vi "Aux TE Controllers Initialization.vi"(8 "Error In":errorcluster, 9 "input cluster":T1={"Loaded Settings File"=path "", "Test Settings"={"Dual Channel"=FALSE, "Air Pump"=FALSE, "Optical Drive"=FALSE, "Pulsed Drive"=FALSE, "Calibration Mode"=FALSE, "Test Sensor ID"=0, "Test Chamber"="", "Test Operator"="", "Sample Descriptor"="", "Notes"=""}, "Calibration Settings"={"Cal. Average"=2, "Cal Averaging"=FALSE, "Tolerance #0"=0.0, "Tolerance #7"=0.0, "Tolerance #6"=0.0, "Tolerance #5"=0.0, "Tolerance #4"=0.0, "Tolerance #3"=0.0, "Tolerance #2"=0.0, "Tolerance #1"=0.0, "Gas Tank Settings"={"Gas Conc. #0"="", "Gas Conc. #1"=0.0, "Gas Conc. #2"=0.0, "Gas Conc. #3"=0.0, "Gas Conc. #4"=0.0, "Gas Conc. #5"=0.0, "Gas Conc. #6"=0.0, "Gas Conc. #7"=0.0}}, "DataLogging Settings"={"Data File Path"=path "c:/data", "Data File Duration (Minutes)"=2.0, "Log Filename"="Test Log.csv", "Config Path"=path ""}, "DAQx Settings"={"DAQ Device"="USBXDAQ", "Frequency"=20.0, "Duty Cycle"=50.0, "Analog Output Settings (Volts)"=[]}, "Capnometer Configuration"={"Serial Port"={"termination char"=10, "End read on termination character?"=TRUE, "Enabled?"=FALSE, "VISA resource name"="COM7", "baud rate"=9600, "data bits"=8, "parity"=enum."None", "stop bits"=10, "flow control"=0, "timeout (ms)"=10000, "Input buffer size"=4096, "End write on termination character?"=FALSE, "XON Char"=17, "XOFF Char"=19}, "Baro Pressure"=760, "Device"=0}, "TE#1 Configuration"={"Temp Set Point"=0.0, "Serial Port"={"termination char"=10, "End read on termination character?"=TRUE, "Enabled?"=FALSE, "VISA resource name"="COM1", "baud rate"=9600, "data bits"=8, "parity"=enum."None", "stop bits"=10, "flow control"=0, "timeout (ms)"=10000, "Input buffer size"=4096, "End write on termination character?"=TRUE, "XON Char"=17, "XOFF Char"=19}}, "TE#2 Configuration"={"Temp Set Point"=0.0, "Serial Port"={"termination char"=10, "End read on termination character?"=TRUE, "Enabled?"=FALSE, "VISA resource name"="COM1", "baud rate"=9600, "data bits"=8, "parity"=enum."None", "stop bits"=10, "flow control"=0, "timeout (ms)"=10000, "Input buffer size"=4096, "End write on termination character?"=TRUE, "XON Char"=17, "XOFF Char"=19}}, "RunTime Mode Settings "={"Resp Rate Brpm "=0.0, "I:E Ratio"=0, "Insp. Gas Tank"=0, "Exp. Gas Tank"=7}, "Chart X axis Timescale"=20, "Pump"=0} {"Pump" items=["Pump 0", "Pump 1", "Pump 2", "Pump 3", "Pump 4", "Pump 5"]; "Chart X axis Timescale" min=20 max=180 step=1; "RunTime Mode Settings"."Exp. Gas Tank" items=["0.07", "0.031", "0.877", "1.863", "3.881", "5.790", "7.688", "6.000"]; "RunTime Mode Settings"."Insp. Gas Tank" items=["0.07", "0.031", "0.877", "1.863", "3.881", "5.790", "7.688", "6.000"]; "RunTime Mode Settings"."I:E Ratio" max=30 scale=0.0..7.0; "RunTime Mode Settings"."Resp Rate Brpm" min=0 max=30 format="%.2f"; "TE#2 Configuration"."Serial Port"."XOFF Char" format="%.0x"; "TE#2 Configuration"."Serial Port"."XON Char" format="%.0x"; "TE#2 Configuration"."Serial Port"."flow control" items=["None"=0, "XON/XOFF"=1, "RTS/CTS"=2, "DTR/DSR"=4]; "TE#2 Configuration"."Serial Port"."stop bits" items=["1.0"=10, "1.5"=15, "2.0"=20]; "TE#2 Configuration"."Serial Port"."data bits" min=5 max=8 step=1; "TE#2 Configuration"."Serial Port"."baud rate" items=["75"=75, "110"=110, "134"=134, "150"=150, "300"=300, "600"=600, "1200"=1200, "1800"=1800, "2400"=2400, "4800"=4800, "7200"=7200, "9600"=9600, "14400"=14400, "19200"=19200, "28800"=28800, "38400"=38400, "56000"=56000, "57600"=57600, "115200"=115200, "128000"=128000, "230400"=230400]; "TE#2 Configuration"."Serial Port"."termination char" format="%.0x"; "TE#1 Configuration"."Serial Port"."XOFF Char" format="%.0x"; "TE#1 Configuration"."Serial Port"."XON Char" format="%.0x"; "TE#1 Configuration"."Serial Port"."flow control" items=["None"=0, "XON/XOFF"=1, "RTS/CTS"=2, "DTR/DSR"=4]; "TE#1 Configuration"."Serial Port"."stop bits" items=["1.0"=10, "1.5"=15, "2.0"=20]; "TE#1 Configuration"."Serial Port"."data bits" min=5 max=8 step=1; "TE#1 Configuration"."Serial Port"."baud rate" items=["75"=75, "110"=110, "134"=134, "150"=150, "300"=300, "600"=600, "1200"=1200, "1800"=1800, "2400"=2400, "4800"=4800, "7200"=7200, "9600"=9600, "14400"=14400, "19200"=19200, "28800"=28800, "38400"=38400, "56000"=56000, "57600"=57600, "115200"=115200, "128000"=128000, "230400"=230400]; "TE#1 Configuration"."Serial Port"."termination char" format="%.0x"; "Capnometer Configuration"."Device" items=["None", "TidalWave", "LoFlow / Canary", "Capnogard"]; "Capnometer Configuration"."Serial Port"."XOFF Char" format="%.0x"; "Capnometer Configuration"."Serial Port"."XON Char" format="%.0x"; "Capnometer Configuration"."Serial Port"."flow control" items=["None"=0, "XON/XOFF"=1, "RTS/CTS"=2, "DTR/DSR"=4]; "Capnometer Configuration"."Serial Port"."stop bits" items=["1.0"=10, "1.5"=15, "2.0"=20]; "Capnometer Configuration"."Serial Port"."data bits" min=5 max=8 step=1; "Capnometer Configuration"."Serial Port"."baud rate" items=["75"=75, "110"=110, "134"=134, "150"=150, "300"=300, "600"=600, "1200"=1200, "1800"=1800, "2400"=2400, "4800"=4800, "7200"=7200, "9600"=9600, "14400"=14400, "19200"=19200, "28800"=28800, "38400"=38400, "56000"=56000, "57600"=57600, "115200"=115200, "128000"=128000, "230400"=230400]; "Capnometer Configuration"."Serial Port"."termination char" format="%.0x"; "DAQx Settings"."Analog Output Settings (Volts)" format="%#.3g"; "DAQx Settings"."Duty Cycle" min=10.0 max=90.0 format="%.1g"; "DAQx Settings"."Frequency" min=20.0 max=200.0; "DataLogging Settings"."Data File Duration (Minutes)" min=2 max=200 format="%#.2g"; "Calibration Settings"."Tolerance #2" min=2 max=4096; "Calibration Settings"."Cal. Average" min=2 max=4096; "Test Settings"."Test Sensor ID" items=["(select)", "RB", "YC", "", "Other"]}) -> (0 "Error Out":errorcluster, 1 "Temp Set Point 2":sgl, 2 "Temp Set Point 1":sgl, 3 "TE Serial Ports Out":T3[](array[typedef]) {"XOFF Char" format="%.0x"; "XON Char" format="%.0x"; "flow control" items=["None"=0, "XON/XOFF"=1, "RTS/CTS"=2, "DTR/DSR"=4]; "stop bits" items=["1.0"=10, "1.5"=15, "2.0"=20]; "data bits" min=5 max=8 step=1; "baud rate" items=["75"=75, "110"=110, "134"=134, "150"=150, "300"=300, "600"=600, "1200"=1200, "1800"=1800, "2400"=2400, "4800"=4800, "7200"=7200, "9600"=9600, "14400"=14400, "19200"=19200, "28800"=28800, "38400"=38400, "56000"=56000, "57600"=57600, "115200"=115200, "128000"=128000, "230400"=230400]; "termination char" format="%.0x"})   [LabVIEW 2016]
uses:
  Controls/Serial Visa Control.ctl
  Controls/UI Settings.ctl
  Controls/Aux CO2 Control.ctl
  Controls/Aux CO2 Selector.ctl
  Controls/Aux TE Control.ctl
  Controls/SerialPortControl.ctl
panel:
  # "Note: Setting Brpm to zero will\ndisable Insp / Exp digital output."
  # "mmHg"
  # "pts"
  # "tolerance"
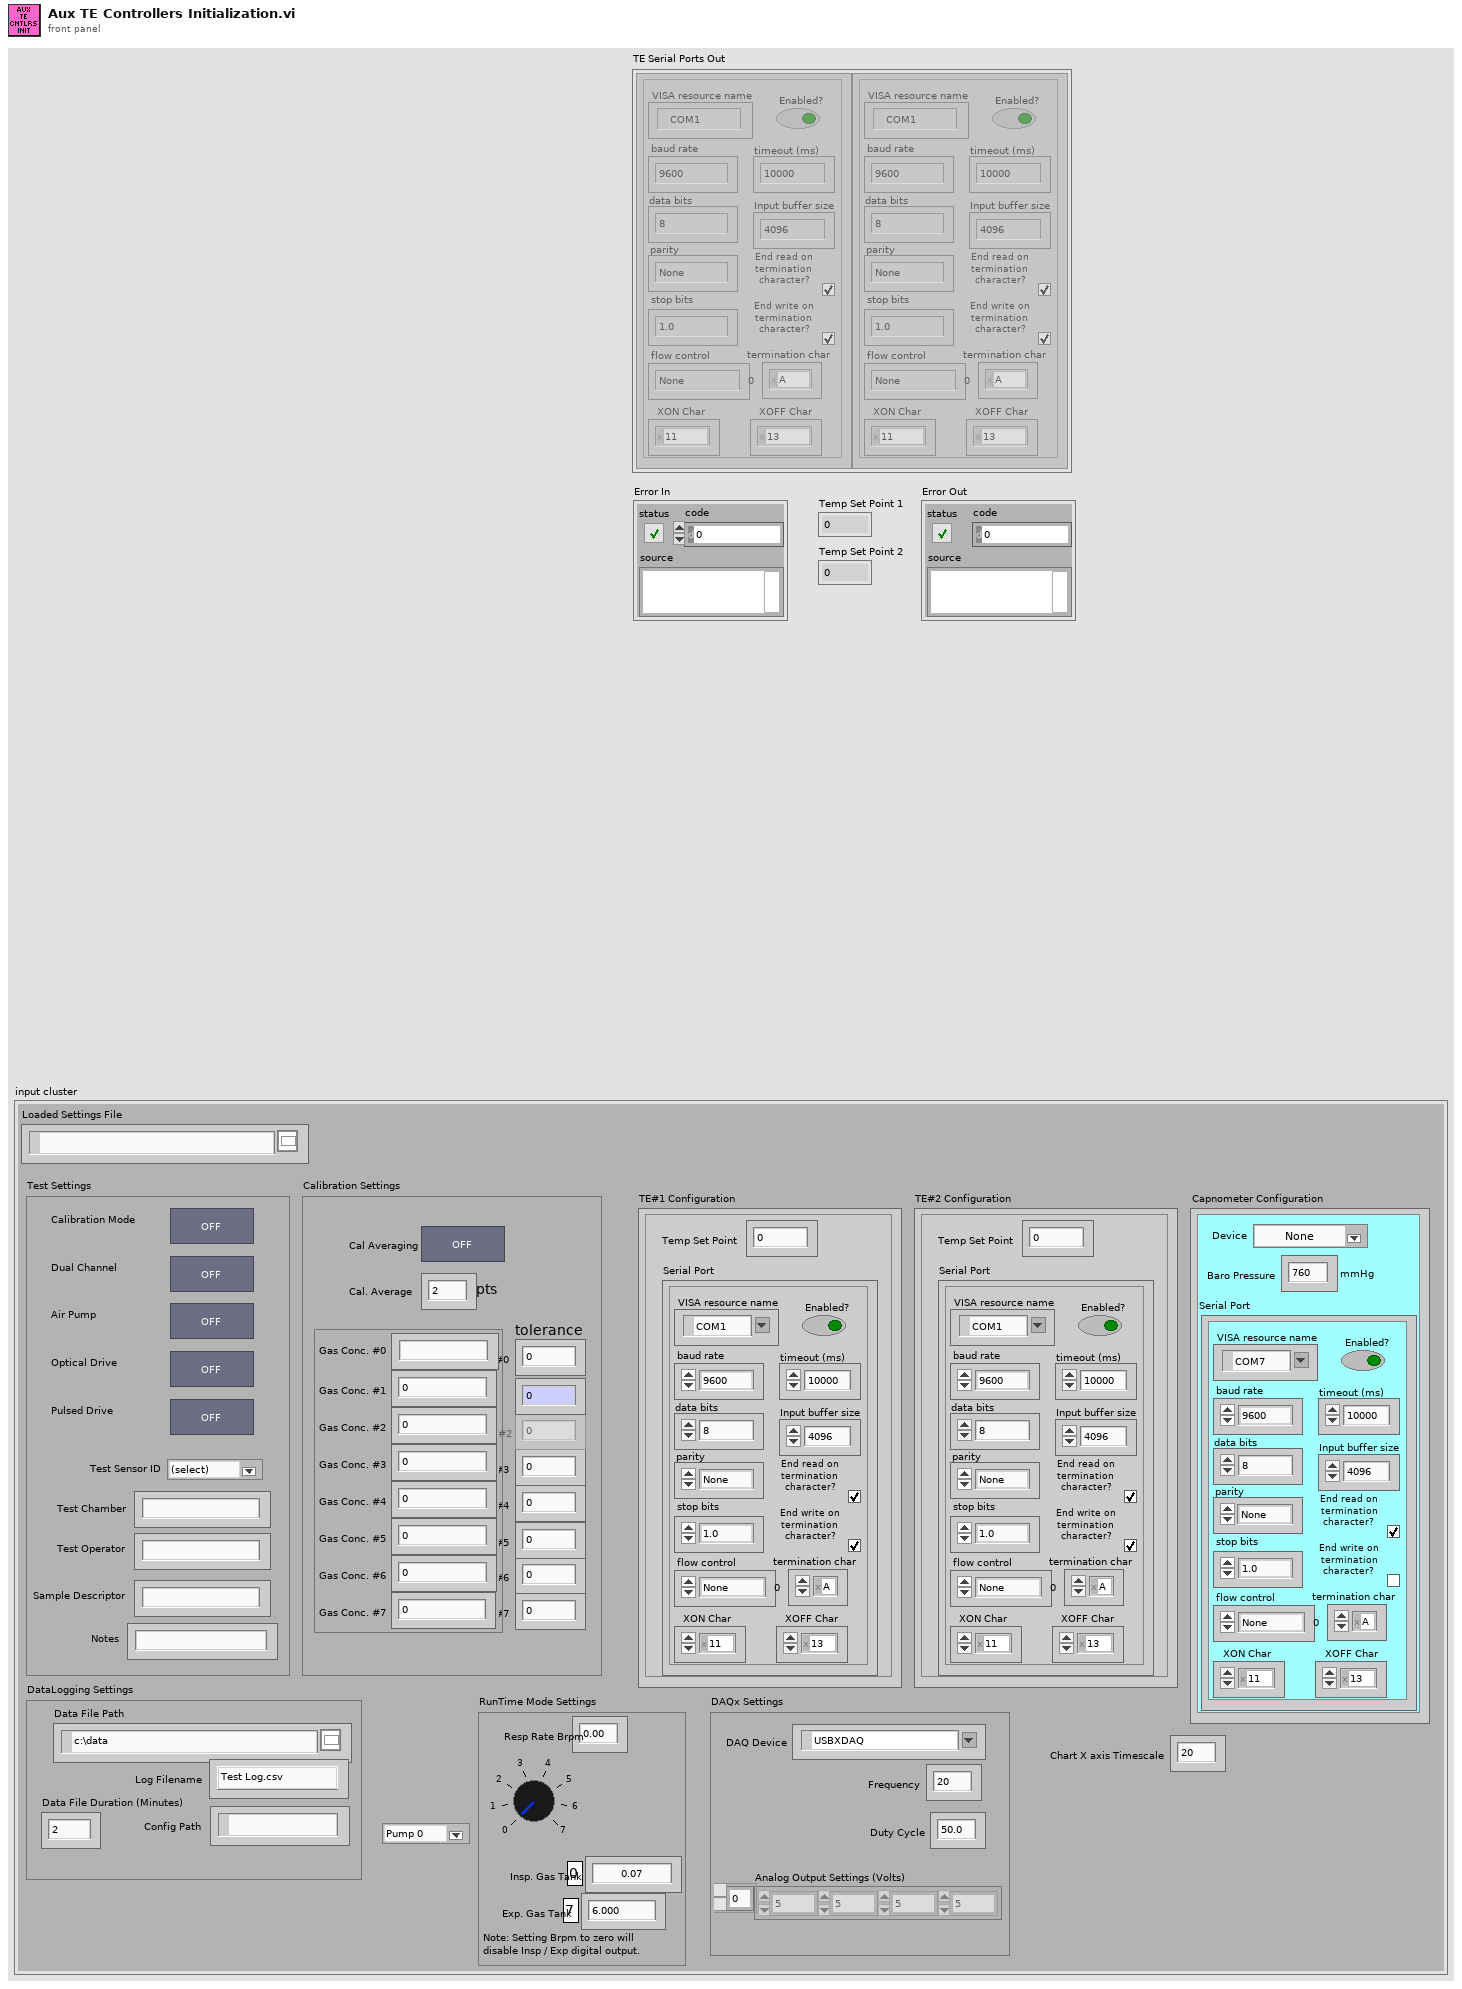
[diagram p1: front panel]
types:
  T1 = typedef "UI Settings.ctl" = cluster{"Loaded Settings File":path, "Test Settings":cluster{"Dual Channel":bool, "Air Pump":bool, "Optical Drive":bool, "Pulsed Drive":bool, "Calibration Mode":bool, "Test Sensor ID":u16, "Test Chamber":string, "Test Operator":string, "Sample Descriptor":string, "Notes":string}, "Calibration Settings":cluster{"Cal. Average":u16, "Cal Averaging":bool, "Tolerance #0":sgl, "Tolerance #7":sgl, "Tolerance #6":sgl, "Tolerance #5":sgl, "Tolerance #4":sgl, "Tolerance #3":sgl, "Tolerance #2":sgl, "Tolerance #1":sgl, "Gas Tank Settings":cluster{"Gas Conc. #0":string, "Gas Conc. #1":sgl, "Gas Conc. #2":sgl, "Gas Conc. #3":sgl, "Gas Conc. #4":sgl, "Gas Conc. #5":sgl, "Gas Conc. #6":sgl, "Gas Conc. #7":sgl}}, "DataLogging Settings":cluster{"Data File Path":path, "Data File Duration (Minutes)":sgl, "Log Filename":string, "Config Path":path}, "DAQx Settings":cluster{"DAQ Device":tag, "Frequency":dbl, "Duty Cycle":dbl, "Analog Output Settings (Volts)":sgl[]}, "Capnometer Configuration":T2, "TE#1 Configuration":T5, "TE#2 Configuration":T5, "RunTime Mode Settings ":cluster{"Resp Rate Brpm ":sgl, "I:E Ratio":u8, "Insp. Gas Tank":u16, "Exp. Gas Tank":u16}, "Chart X axis Timescale":u16, "Pump":u16}
  T2 = typedef "Aux CO2 Control.ctl" = cluster{"Serial Port":T3, "Baro Pressure":u32, "Device":T4}
  T3 = typedef "Serial Visa Control.ctl" = cluster{"termination char":u8, "End read on termination character?":bool, "Enabled?":bool, "VISA resource name":refnum<visa-resource-name>, "baud rate":u32, "data bits":u16, "parity":enum16{"None", "Odd", "Even", "Mark", "Space"}, "stop bits":u16, "flow control":u16, "timeout (ms)":u32, "Input buffer size":u32, "End write on termination character?":bool, "XON Char":u8, "XOFF Char":u8}
  T4 = typedef "Aux CO2 Selector.ctl" = u16
  T5 = typedef "Aux TE Control.ctl" = cluster{"Temp Set Point":sgl, "Serial Port":T3}
  T6 = typedef "SerialPortControl.ctl" = enum16{"Initialize", "Write Data", "Read Data", "Close Port"}
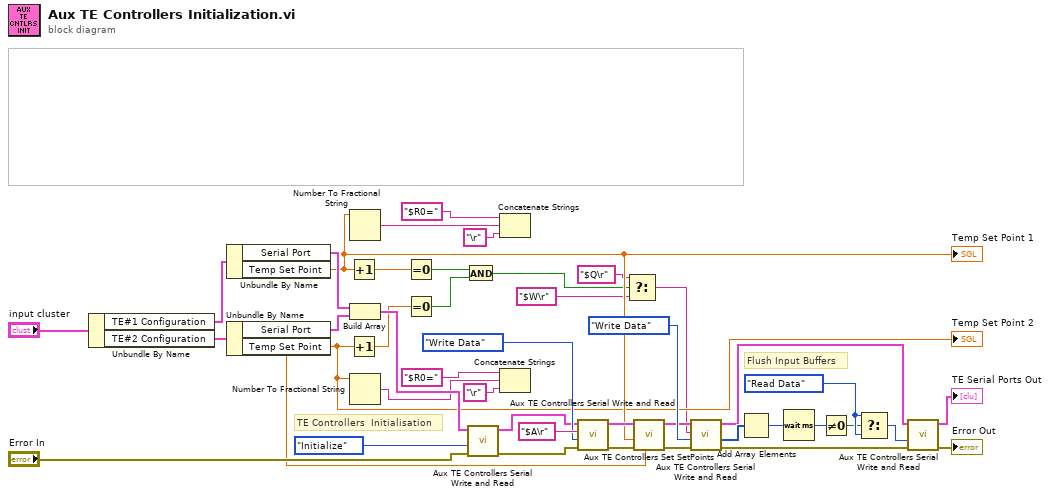
[diagram p0: block diagram]
diagram:
  w23 = SerialPortControl."Read Data" ("Action")
  # "Flush Input Buffers"
  # "TE Controllers  Initialisation"
  n1 = Unbundle By Name("input cluster") -> ("TE#1 Configuration"=w2:T5, "TE#2 Configuration"=w1:T5)
  n2 = Unbundle By Name(w2) -> ("Serial Port"=w40:T3, "Temp Set Point"=w12:sgl)
  "Temp Set Point 1" <- w12
  n3 = Unbundle By Name(w1) -> ("Serial Port"=w39:T3, "Temp Set Point"=w10:sgl)
  "Temp Set Point 2" <- w10
  n4 = Increment(x=w12) -> (x+1=w13:sgl)
  n5 = Increment(x=w10) -> (x+1=w11:sgl)
  n6 = Number To Fractional String(number=w12) -> (F-format string=w37:string)  [unwired: 3 in]
  n7 = Build Array(w40, w39) -> (w42:T3[])
  n8 = Number To Fractional String(number=w10) -> (F-format string=w26:string)  [unwired: 3 in]
  n9 = Equal To 0?(x=w13) -> (x = 0?=w8:bool)
  n10 = Equal To 0?(x=w11) -> (x = 0?=w9:bool)
  n11 = And(x=w8, y=w9) -> (x .and. y?=w7:bool)
  n12 = call "Aux TE Controllers Serial Write and Read.vi"("error in"="Error In", "Action"=SerialPortControl."Initialize", "TE Controller Serial Ports In"=w42) -> ("Error Out"=w19:errorcluster, "TE Controller Serial Ports Out"=w18:T3[])  [unwired: 2 in, 3 out]
  n13 = Concatenate Strings("$R0=" ("string to write"), w37, "\r" ("string to write")) -> ()  [unwired: 1 out]
  n14 = Concatenate Strings("$R0=" ("string to write"), w26, "\r" ("string to write")) -> ()  [unwired: 1 out]
  n15 = call "Aux TE Controllers Serial Write and Read.vi"("error in"=w19, "Action"=SerialPortControl."Write Data", "string to write"="$A\r", "TE Controller Serial Ports In"=w18) -> ("Error Out"=w15:errorcluster, "TE Controller Serial Ports Out"=w14:T3[])  [unwired: 1 in, 3 out]
  n16 = Select(t="$Q\r" ("string to write"), s=w7, f="$W\r" ("string to write")) -> (s? t:f=w5:string)
  n17 = call "Aux TE Controllers Set SetPoints.vi"("Set Point2"=w10, "Error In"=w15, "Set Point1"=w12, "TE Serial Ports In"=w14) -> ("Error Out"=w16:errorcluster, "TE Serial Ports Out"=w17:T3[])  [unwired: 5 in, 1 out]
  n18 = call "Aux TE Controllers Serial Write and Read.vi"("error in"=w16, "Action"=SerialPortControl."Write Data", "string to write"=w5, "TE Controller Serial Ports In"=w17) -> ("Error Out"=w30:errorcluster, "#Bytes R/W"=w34:i16[], "TE Controller Serial Ports Out"=w31:T3[])  [unwired: 1 in, 2 out]
  n19 = Add Array Elements(numeric array=w34) -> (sum=w33:i16)
  n20 = Wait (ms)(milliseconds to wait=w33) -> (millisecond timer value=w32:u32)
  n21 = Not Equal To 0?(x=w32) -> (x != 0?=w22:bool)
  n22 = Select(t=w23, s=w22, f=w23) -> (s? t:f=w24:T6)
  n23 = call "Aux TE Controllers Serial Write and Read.vi"("error in"=w30, "Action"=w24, "TE Controller Serial Ports In"=w31) -> ("Error Out"=→"Error Out":errorcluster, "TE Controller Serial Ports Out"=→"TE Serial Ports Out":T3[])  [unwired: 2 in, 3 out]
